vi "Read Current Laser Power.vi"(8 "error in (no error)":errorcluster, 11 "Sim Laser Driver in":refnum<class "Sim Laser Driver.lvclass">) -> (0 "error out":errorcluster, 2 "Current Laser Power":dbl, 3 "Sim Laser Driver out":refnum<class "Sim Laser Driver.lvclass">)   [LabVIEW 2022 SP3, in "Sim Laser Driver.lvclass"]
uses:
  Sim Laser Driver.lvclass
  Sim Laser Driver.lvclass/Sim Laser Driver.ctl
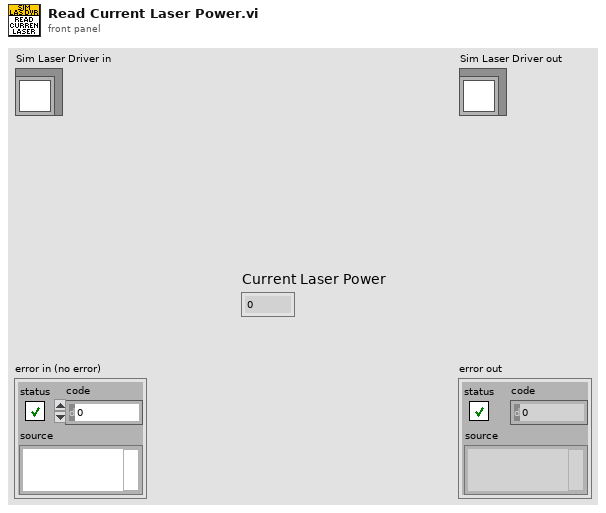
[diagram p1: front panel]
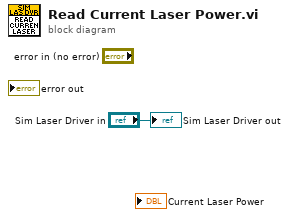
[diagram p0: block diagram]
diagram:
  "Sim Laser Driver out" <- "Sim Laser Driver in"
